vi "ConvertTime.vi"(11 "Час1":dbl) -> (0 "Минути":dbl, 3 "Час":i64)   [LabVIEW 2023]
panel:
  out "x-y":dbl format="%#_8g"
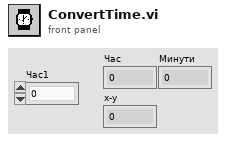
[diagram p1: front panel]
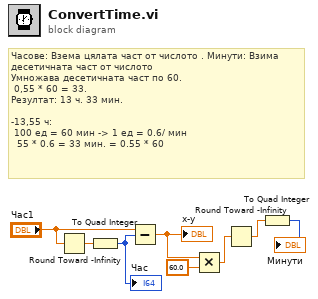
[diagram p0: block diagram]
diagram:
  # "Часове: Взема цялата част от числото . Минути: Взима десетичната част от числото \nУмножава десетичната част по 60. \n 0,55 * 60 = 33.\nРезултат: 13 ч. 33 мин.\n\n-13,55 ч: \n 100 ед = 60 мин -> 1 ед = 0.6/ мин \n  55 * 0.6 = 33 мин. = 0.55 * 60"
  n1 = Round Toward -Infinity(1:"Час1") -> (0:w8:dbl)
  n2 = To Quad Integer(1:w8) -> (0:w7:i64)
  "Час" <- w7
  n3 = Subtract(x="Час1", y=w7) -> (x-y=w5:dbl)
  "x-y" <- w5
  n4 = Multiply(x=w5, y=60.0) -> (x*y=w2:dbl)
  n5 = Round Toward -Infinity(1:w2) -> (0:w1:dbl)
  n6 = To Quad Integer(1:w1) -> (0:→"Минути":i64)
